vi "ReverseWaveforms.vi"(11 "signal(s) in":waveform(dbl)[](array[waveform])=[{"t0"=timestamp(0 s since 1904-01-01), "dt"=5e-05, "Y"=array[2399 elements]}, {"t0"=timestamp(0 s since 1904-01-01), "dt"=5e-05, "Y"=array[2399 elements]}]) -> (3 "signal(s) out":waveform(dbl)[](array[waveform]))   [LabVIEW 2015]
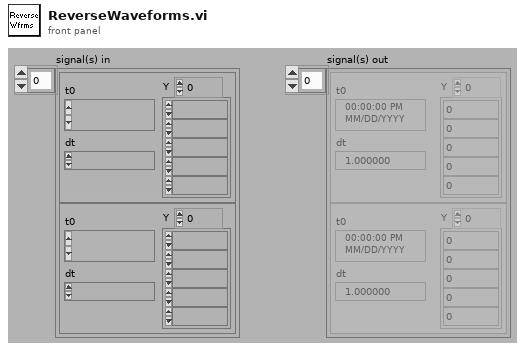
[diagram p1: front panel]
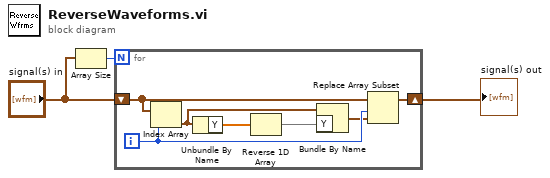
[diagram p0: block diagram]
diagram:
  n1 = Array Size(array="signal(s) in") -> (size(s)=w3:i32)
  n2 = for {
    N: w3 -> [_]
    shift-right: [w6] -> w1
    shift-left: "signal(s) in" -> [w7]
    i -> [w9]
    n3 = Index Array(array=w7, index=w9) -> (element=w4:waveform(dbl))
    n4 = Unbundle By Name(w4) -> ("Y"=w10:dbl[])
    n5 = Reverse 1D Array(array=w10) -> (reversed array=w5:dbl[])
    n6 = Bundle By Name(cluster=w4, "Y"=w5) -> (w8:waveform(dbl))
    n7 = Replace Array Subset(array=w7, new element=w8, index=w9) -> (w6:waveform(dbl)[])
  }
  "signal(s) out" <- w1
